vi "PC Controller.vi"() -> ()   [LabVIEW 2017]
panel:
  out "Previous System Status":string
  out "TCP Error Code":i8
  out "Recieved from MyRIO":dbl
  out "TCP Stop Latch":bool
  in  "Send to MyRIO":dbl
  out "System Status":string
  in  "System switch":bool
  in  "MyRIO IP Address":string="localhost"
  out "Current Time":timestamp format="%<%H:%M:%S\n%x>T"
  in  "Logout":bool
  out "Close Event 4 LED":bool
  out "Open Event 4 LED":bool
  out "Close Event 3 LED":bool
  out "Open Event 3 LED":bool
  in  "Close Event Time 4 Edit":timestamp format="%<%H:%M:%S\n%x>T"
  in  "Open Event Time 4 Edit":timestamp format="%<%H:%M:%S\n%x>T"
  in  "Close Event Time 3 Edit":timestamp format="%<%H:%M:%S\n%x>T"
  in  "Open Event Time 3 Edit":timestamp format="%<%H:%M:%S\n%x>T"
  out "Close Event Time 4":timestamp format="%<%H:%M:%S\n%x>T"
  out "Open Event Time 4":timestamp format="%<%H:%M:%S\n%x>T"
  out "Close Event Time 3":timestamp format="%<%H:%M:%S\n%x>T"
  out "Open Event Time 3":timestamp format="%<%H:%M:%S\n%x>T"
  out "Close Event 2 LED":bool
  out "Open Event 2 LED":bool
  out "Close Event 1 LED":bool
  out "Open Event 1 LED":bool
  in  "Close Event Time 2 Edit":timestamp format="%<%H:%M:%S\n%x>T"
  in  "Open Event Time 2 Edit":timestamp format="%<%H:%M:%S\n%x>T"
  in  "Close Event Time 1 Edit":timestamp format="%<%H:%M:%S\n%x>T"
  in  "Open Event Time 1 Edit":timestamp format="%<%H:%M:%S\n%x>T"
  out "Close Event Time 2":timestamp format="%<%H:%M:%S\n%x>T"
  out "Open Event Time 2":timestamp format="%<%H:%M:%S\n%x>T"
  out "Close Event Time 1":timestamp format="%<%H:%M:%S\n%x>T"
  out "Open Event Time 1":timestamp format="%<%H:%M:%S\n%x>T"
  out "Login Attempts":i8
  out "Login Status":string
  in  "Login Button":bool
  in  "Password":string
  in  "Username":string
  out "MyRIO Movement":T1(graph)
  out "Core Temp":dbl format="%#_4g"
  # "Event Time"
  # "Status"
  # "Change Event Time"
  # "On"
  # "Off"
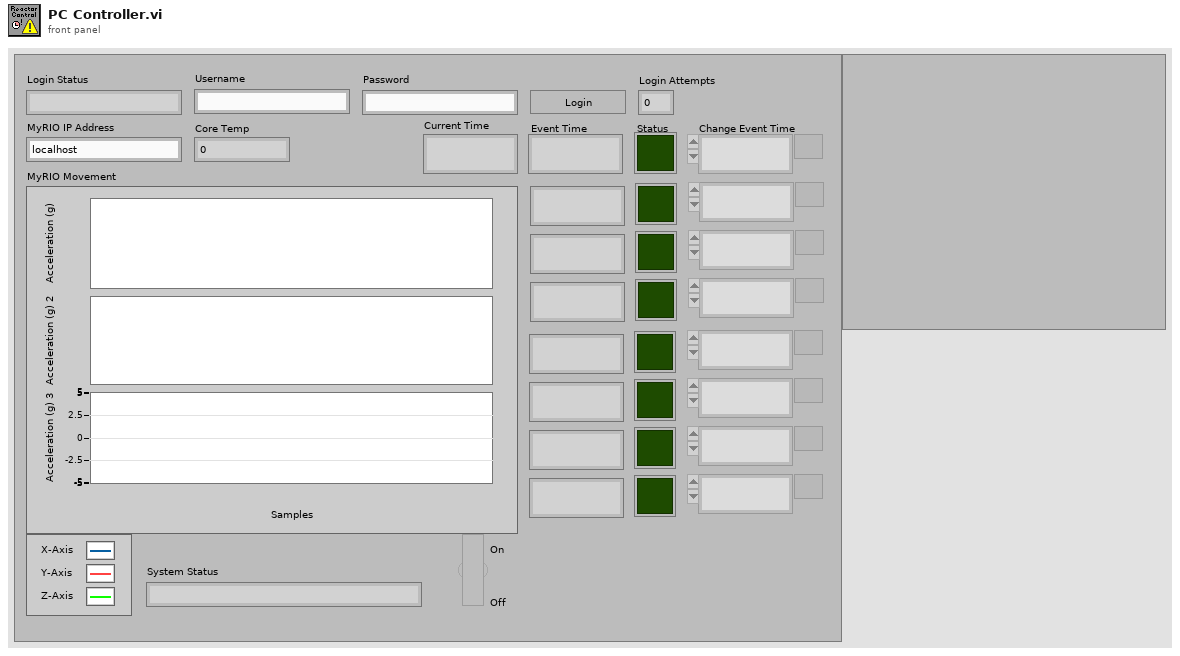
[diagram p1: front panel]
types:
  T1 = cluster{"X-Axis":dbl, "Y-Axis":dbl, "Z-Axis":dbl}
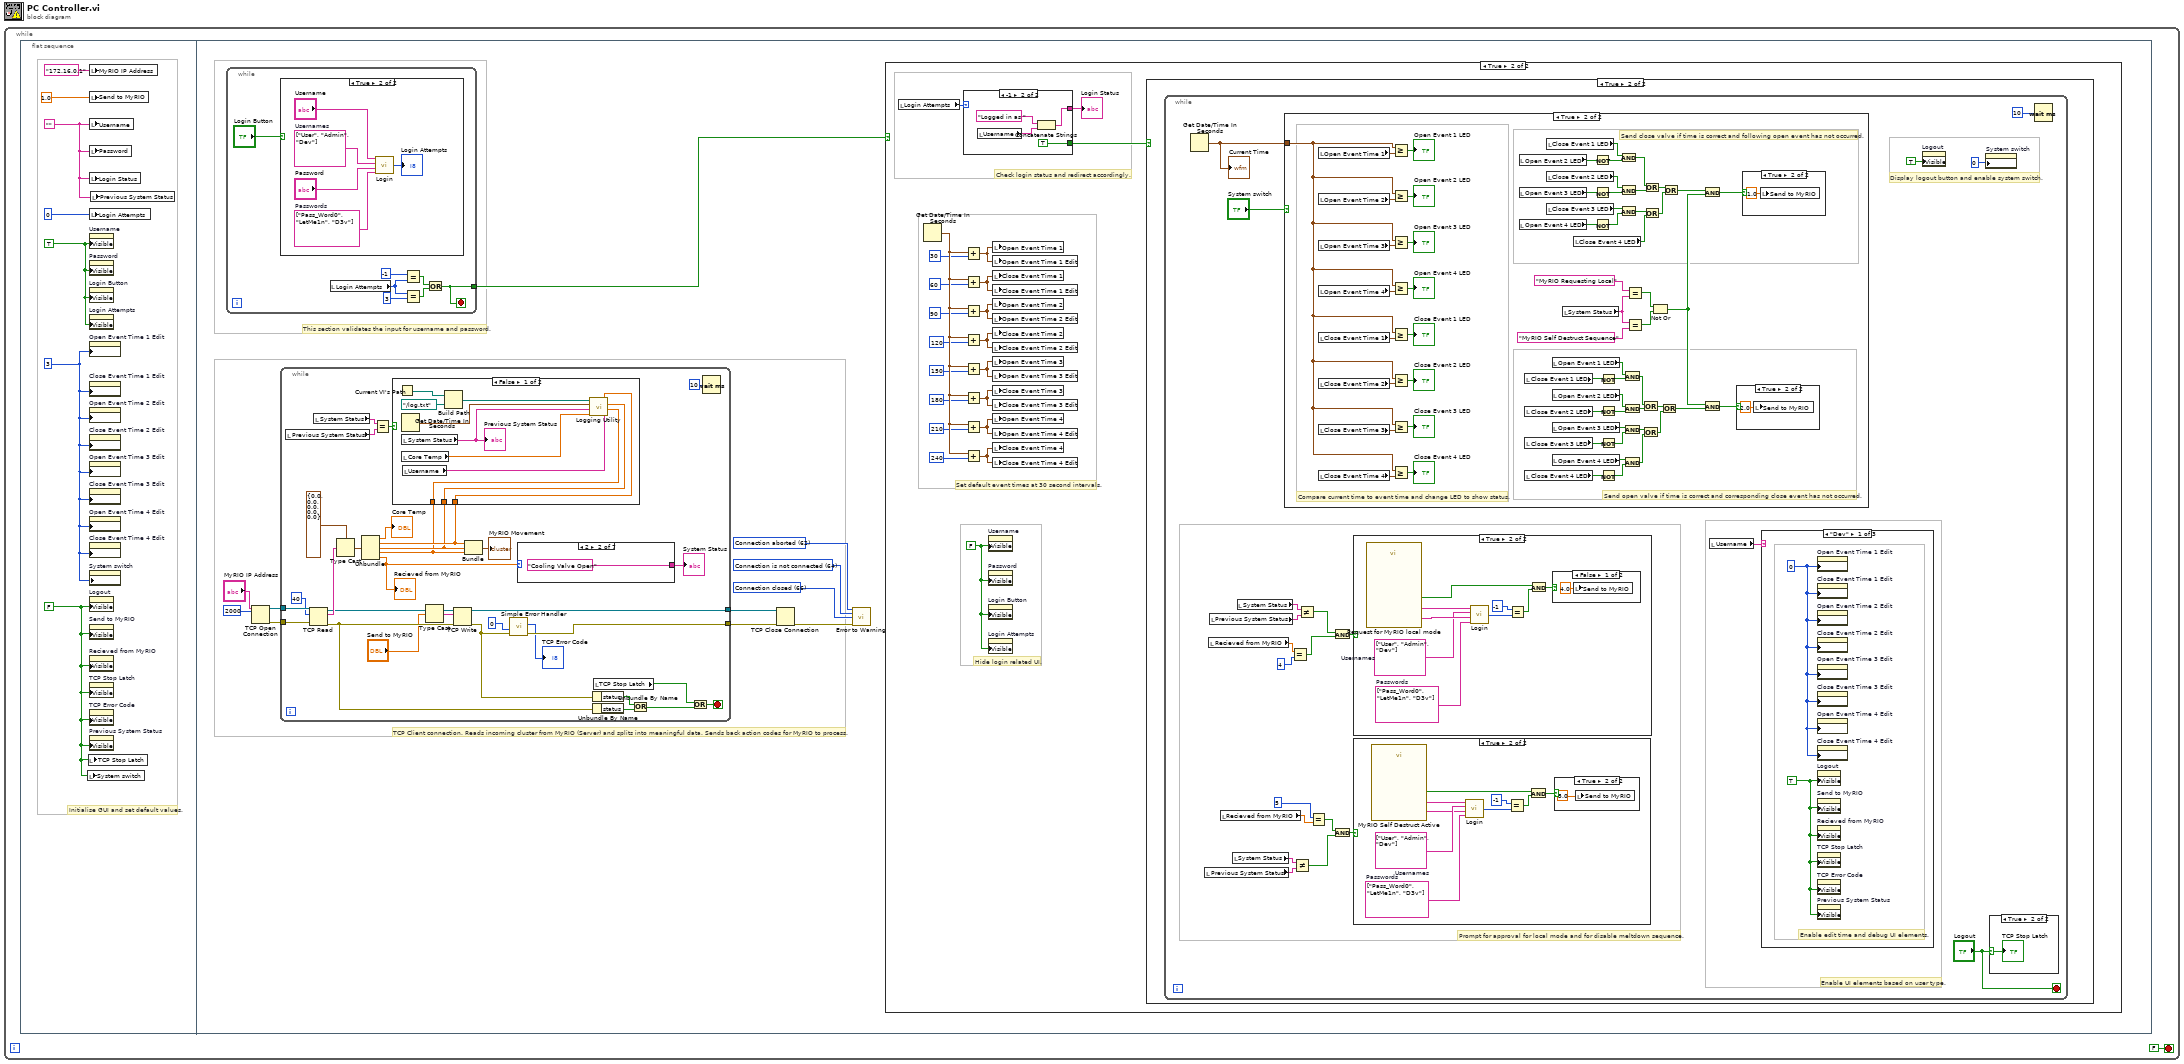
[diagram p0: block diagram]
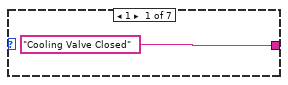
[diagram p3: hidden frame]
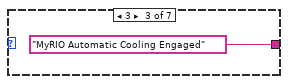
[diagram p4: hidden frame]
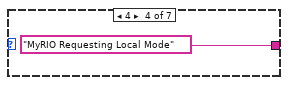
[diagram p5: hidden frame]
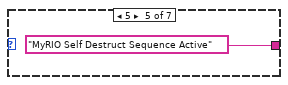
[diagram p6: hidden frame]
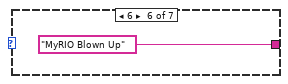
[diagram p7: hidden frame]
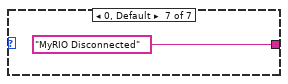
[diagram p8: hidden frame]
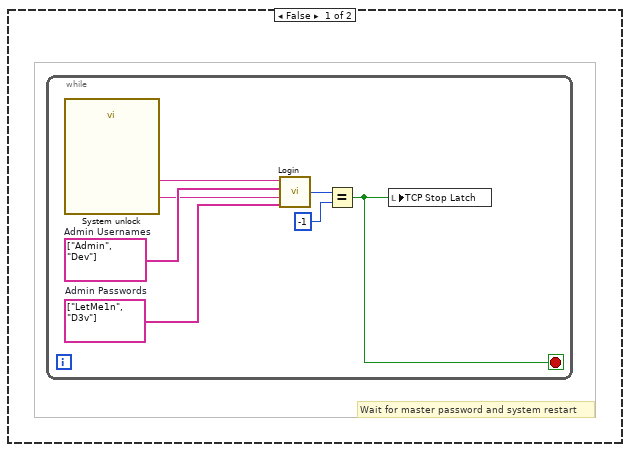
[diagram p10: hidden frame]
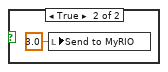
[diagram p14: hidden frame]
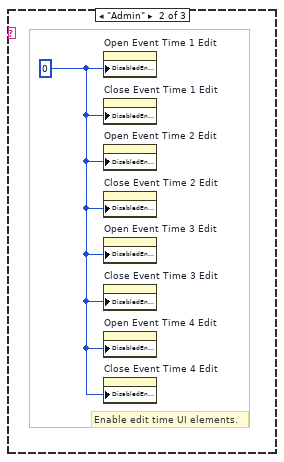
[diagram p15: hidden frame]
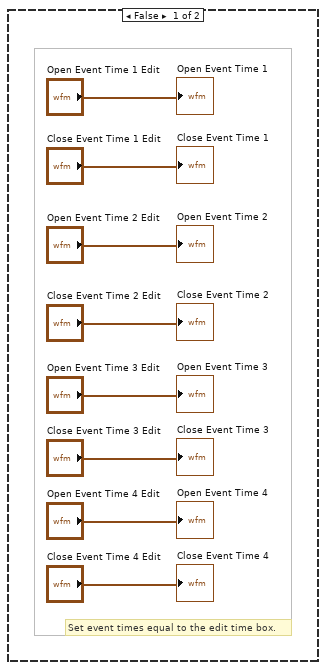
[diagram p17: hidden frame]
diagram:
  n1 = while {
    stop <- FALSE stop-if-true
    n2 = flat-sequence {
      frame #0 {
        w3 = FALSE
        w8 = TRUE
        w7 = 3
        w2 = ""
        # "Initialise GUI and set default values."
        n3 = local write "System switch"(w3) -> ()
        n4 = local write "TCP Stop Latch"(w3) -> ()
        n5 = local write "MyRIO IP Address"("172.16.0.1") -> ()
        n6 = local write "Send to MyRIO"(1.0) -> ()
        n7 = local write "Username"(w2) -> ()
        n8 = local write "Password"(w2) -> ()
        n9 = local write "Login Status"(w2) -> ()
        n10 = local write "Login Attempts"(u32 0 ("milliseconds to wait")) -> ()
        n11 = property on="Username" class="Str"("Visible"=w8) -> ()  [unwired: 2 in, 2 out]
        n12 = property on="Password" class="Str"("Visible"=w8) -> ()  [unwired: 2 in, 2 out]
        n13 = property on="Login Button" class="Bool"("Visible"=w8) -> ()  [unwired: 2 in, 2 out]
        n14 = property on="Login Attempts" class="DigNum (strict)"("Visible"=w8) -> ()  [unwired: 2 in, 2 out]
        n15 = property on="Open Event Time 1 Edit" class="AbsTime (strict)"("DisabledEnum"=w7) -> ()  [unwired: 2 in, 2 out]
        n16 = property on="Close Event Time 1 Edit" class="AbsTime (strict)"("DisabledEnum"=w7) -> ()  [unwired: 2 in, 2 out]
        n17 = property on="Open Event Time 2 Edit" class="AbsTime (strict)"("DisabledEnum"=w7) -> ()  [unwired: 2 in, 2 out]
        n18 = property on="Close Event Time 2 Edit" class="AbsTime (strict)"("DisabledEnum"=w7) -> ()  [unwired: 2 in, 2 out]
        n19 = property on="Open Event Time 3 Edit" class="AbsTime (strict)"("DisabledEnum"=w7) -> ()  [unwired: 2 in, 2 out]
        n20 = property on="Close Event Time 3 Edit" class="AbsTime (strict)"("DisabledEnum"=w7) -> ()  [unwired: 2 in, 2 out]
        n21 = property on="Open Event Time 4 Edit" class="AbsTime (strict)"("DisabledEnum"=w7) -> ()  [unwired: 2 in, 2 out]
        n22 = property on="Close Event Time 4 Edit" class="AbsTime (strict)"("DisabledEnum"=w7) -> ()  [unwired: 2 in, 2 out]
        n23 = property on="Logout" class="Bool"("Visible"=w3) -> ()  [unwired: 2 in, 2 out]
        n24 = property on="Send to MyRIO" class="DigNum (strict)"("Visible"=w3) -> ()  [unwired: 2 in, 2 out]
        n25 = property on="Recieved from MyRIO" class="DigNum (strict)"("Visible"=w3) -> ()  [unwired: 2 in, 2 out]
        n26 = property on="TCP Stop Latch" class="Bool (strict)"("Visible"=w3) -> ()  [unwired: 2 in, 2 out]
        n27 = property on="TCP Error Code" class="DigNum (strict)"("Visible"=w3) -> ()  [unwired: 2 in, 2 out]
        n28 = property on="Previous System Status" class="Str"("Visible"=w3) -> ()  [unwired: 2 in, 2 out]
        n29 = property on="System switch" class="Bool (strict)"("DisabledEnum"=w7) -> ()  [unwired: 2 in, 2 out]
        n30 = local write "Previous System Status"(w2) -> ()
      }
      frame #1 {
        w9 = 66 items=["No Error", "Argument Error", "Memory Full", "Out of Zone", "End of File", "File Already Open", "Generic File IO Error", "File Not Found", "File Permission Error", "Disk Full", "Duplicate Path", "Too Many Files Open", "Not Enabled", "Resource File Not Found", "Cannot Add Resource", "Resource Not Found", "Image Not Found", "Image Memory Error", "Pen Does Not Exist", "Config Bad Type", "Config Token Not Found", "Config Parse Error", "Config Memory Error", "Bad External Code Format", "Bad External Code Offset", "External Code Not Present", "Null Window", "Destroy Window Mixup", "Null Menu", "Print Aborted", "Bad Print Record", "Print Driver Error", "Windows Error During Print", "Memory Error During Print", "Print Dialog Error", "Generic Print Error", "Invalid Device Refnum", "Device Not Found", "Device Parameter Error", "Device Unit Error", "Can't Open Device", "Device Call Aborted", "Generic Error", "Cancelled By User", "Object ID Too Low", "Object ID Too High", "Object Not In Heap", "Unknown Heap", "Bad DefProc ID", "DefProc Not In Table", "Message Out Of Range", "Null Method", "Unknown Message", "Manager Call Not Supported", "Bad address", "Connection In progress", "Connection timed out", "Connection is already in progress", "Network attribute not supported", "Network error", "Address in use", "System out of memory", "Connection aborted", "Connection refused", "Connection is not connected", "Connection is already connected", "Connection closed", "Initialize error (interapplication manager)", "Bad occurrence", "Wait on unbound occurrence handler", "Occurrence queue overflow", "Bad path", "Semaphore not signaled", "Unrecognized type (interapplication manager)"] ("1st Error to Convert")
        w10 = 64 items=["No Error", "Argument Error", "Memory Full", "Out of Zone", "End of File", "File Already Open", "Generic File IO Error", "File Not Found", "File Permission Error", "Disk Full", "Duplicate Path", "Too Many Files Open", "Not Enabled", "Resource File Not Found", "Cannot Add Resource", "Resource Not Found", "Image Not Found", "Image Memory Error", "Pen Does Not Exist", "Config Bad Type", "Config Token Not Found", "Config Parse Error", "Config Memory Error", "Bad External Code Format", "Bad External Code Offset", "External Code Not Present", "Null Window", "Destroy Window Mixup", "Null Menu", "Print Aborted", "Bad Print Record", "Print Driver Error", "Windows Error During Print", "Memory Error During Print", "Print Dialog Error", "Generic Print Error", "Invalid Device Refnum", "Device Not Found", "Device Parameter Error", "Device Unit Error", "Can't Open Device", "Device Call Aborted", "Generic Error", "Cancelled By User", "Object ID Too Low", "Object ID Too High", "Object Not In Heap", "Unknown Heap", "Bad DefProc ID", "DefProc Not In Table", "Message Out Of Range", "Null Method", "Unknown Message", "Manager Call Not Supported", "Bad address", "Connection In progress", "Connection timed out", "Connection is already in progress", "Network attribute not supported", "Network error", "Address in use", "System out of memory", "Connection aborted", "Connection refused", "Connection is not connected", "Connection is already connected", "Connection closed", "Initialize error (interapplication manager)", "Bad occurrence", "Wait on unbound occurrence handler", "Occurrence queue overflow", "Bad path", "Semaphore not signaled", "Unrecognized type (interapplication manager)"] ("1st Error to Convert")
        w11 = 62 items=["No Error", "Argument Error", "Memory Full", "Out of Zone", "End of File", "File Already Open", "Generic File IO Error", "File Not Found", "File Permission Error", "Disk Full", "Duplicate Path", "Too Many Files Open", "Not Enabled", "Resource File Not Found", "Cannot Add Resource", "Resource Not Found", "Image Not Found", "Image Memory Error", "Pen Does Not Exist", "Config Bad Type", "Config Token Not Found", "Config Parse Error", "Config Memory Error", "Bad External Code Format", "Bad External Code Offset", "External Code Not Present", "Null Window", "Destroy Window Mixup", "Null Menu", "Print Aborted", "Bad Print Record", "Print Driver Error", "Windows Error During Print", "Memory Error During Print", "Print Dialog Error", "Generic Print Error", "Invalid Device Refnum", "Device Not Found", "Device Parameter Error", "Device Unit Error", "Can't Open Device", "Device Call Aborted", "Generic Error", "Cancelled By User", "Object ID Too Low", "Object ID Too High", "Object Not In Heap", "Unknown Heap", "Bad DefProc ID", "DefProc Not In Table", "Message Out Of Range", "Null Method", "Unknown Message", "Manager Call Not Supported", "Bad address", "Connection In progress", "Connection timed out", "Connection is already in progress", "Network attribute not supported", "Network error", "Address in use", "System out of memory", "Connection aborted", "Connection refused", "Connection is not connected", "Connection is already connected", "Connection closed", "Initialize error (interapplication manager)", "Bad occurrence", "Wait on unbound occurrence handler", "Occurrence queue overflow", "Bad path", "Semaphore not signaled", "Unrecognized type (interapplication manager)"] ("1st Error to Convert")
        # "TCP Client connection. Reads incoming cluster from MyRIO (Server) and splits into meaningful data. Sends back action codes for MyRIO to process."
        # "This section validates the input for username and password."
        n31 = while {
          tunnel: [w218] -> w19
          stop <- w218 stop-if-true
          n32 = case shown="True" "Login Button" {
            frame False {
            }
            frame True {
              w226 = string[] ["Pass_Word0", "LetMe1n", "D3v"]  # Passwords
              w228 = string[] ["User", "Admin", "Dev"]  # Usernames
              n33 = call "Login.vi"("Passwords"=w226, "Password"="Password", "Usernames"=w228, "Username"="Username") -> ("Login Attempts"=→"Login Attempts":i8)
            }
          }
          n34 = local read "Login Attempts"() -> (w221:i8)
          n35 = Equal?(x=-1, y=w221) -> (x = y?=w220:bool)
          n36 = Equal?(x=w221, y=3) -> (x = y?=w219:bool)
          n37 = Or(x=w220, y=w219) -> (x .or. y?=w218:bool)
        }
        n38 = TCP Open Connection(address="MyRIO IP Address", remote port or service name=u16 2000) -> (connection ID=w14:refnum<k5>, error out=w15:errorcluster)  [unwired: 1 in, 2 out]
        n39 = while {
          tunnel: w15 -> [w50]
          tunnel: w14 -> [w49]
          tunnel: [w32] -> w17
          tunnel: [w33] -> w18
          stop <- w37 stop-if-true
          n40 = local read "Previous System Status"() -> (w25:string)
          n41 = TCP Read(connection ID=w49, bytes to read=40, error in (no error)=w50) -> (connection ID out=w42:refnum<k5>, data out=w47:string, error out=w41:errorcluster)  [unwired: 2 in]
          n42 = local read "System Status"() -> (w26:string)
          n43 = Type Cast(type=cluster{dbl, dbl, dbl, dbl, dbl} {0.0, 0.0, 0.0, 0.0, 0.0}, x=w47) -> (*(type *) &x=w45:cluster{dbl, dbl, dbl, dbl, dbl})
          n44 = Unbundle(w45) -> (→"Core Temp":dbl, w22:dbl, w21:dbl, w20:dbl, w27:dbl)
          "Recieved from MyRIO" <- w27
          n45 = Equal?(x=w26, y=w25) -> (x = y?=w24:bool)
          n46 = case shown="False" w24 {
            tunnel: w22 -> [w53 _]
            tunnel: w21 -> [w52 _]
            tunnel: w20 -> [w51 _]
            frame False {
              n47 = Current VI's Path() -> (path=w60:path)
              n48 = Get Date/Time In Seconds() -> (seconds since 1Jan1904=w55:timestamp)
              n49 = local read "System Status"() -> (w57:string)
              "Previous System Status" <- w57
              n50 = local read "Core Temp"() -> (w54:dbl)
              n51 = local read "Username"() -> (w56:string)
              n52 = Build Path(base path=w60, name or relative path=path "../log.txt") -> (appended path=w58:path)
              n53 = call "Logging Utility.vi"("Username"=w56, "Z Coord"=w51, "Y Coord"=w52, "X Coord"=w53, "Temperature"=w54, "Event"=w57, "Timestamp"=w55, "Path"=w58) -> ()
            }
            frame True {
            }
          }
          n54 = Type Cast(x="Send to MyRIO") -> (*(type *) &x=w40:string)  [unwired: 1 in]
          n55 = TCP Write(connection ID=w42, data in=w40, error in (no error)=w41) -> (connection ID out=w33:refnum<k5>, error out=w31:errorcluster)  [unwired: 1 in, 1 out]
          n56 = Bundle(w22, w21, w20) -> (→"MyRIO Movement":cluster{dbl, dbl, dbl})  [unwired: 1 in]
          n57 = call <vilib>:"Simple Error Handler.vi"("type of dialog (OK msg:1)"=u32 0 ("milliseconds to wait"), "error in (no error)"=w31) -> ("code out"=→"TCP Error Code":i32, "error out"=w32:errorcluster)  [unwired: 3 in, 3 out]
          n58 = case shown="2" w27 {
            tunnel: ["Cooling Valve Closed" "Cooling Valve Open" "MyRIO Automatic Cooling Engaged" "MyRIO Requesting Local Mode" "MyRIO Self Destruct Sequence Active" "MyRIO Blown Up" "MyRIO Disconnected"] -> w28
            frame 1 {
            }
            frame 2 {
            }
            frame 3 {
            }
            frame 4 {
            }
            frame 5 {
            }
            frame 6 {
            }
            frame 0, Default {
            }
          }
          "System Status" <- w28
          n59 = Unbundle By Name(w31) -> ("status"=w38:bool)
          n60 = Unbundle By Name(w41) -> ("status"=w39:bool)
          n61 = local read "TCP Stop Latch"() -> (w35:bool)
          n62 = Or(x=w38, y=w39) -> (x .or. y?=w36:bool)
          n63 = Or(x=w35, y=w36) -> (x .or. y?=w37:bool)
          n64 = Wait (ms)(milliseconds to wait=u32 10) -> ()  [unwired: 1 out]
        }
        n65 = TCP Close Connection(connection ID=w18, error in (no error)=w17) -> (error out=w12:errorcluster)  [unwired: 1 in, 1 out]
        n66 = call <vilib>:"Error to Warning.vi"("1st Error to Convert"=w11, "2nd Error to Convert"=w10, "3rd Error to Convert"=w9, "error in"=w12) -> ()  [unwired: 2 in, 10 out]
        n67 = case shown="True" w19 {
          frame False {
          }
          frame True {
            w86 = FALSE
            # "Set default event times at 30 second intervals."
            # "Hide login related UI."
            # "Check login status and redirect accordingly."
            n68 = local read "Login Attempts"() -> (w88:i8)
            n69 = Get Date/Time In Seconds() -> (seconds since 1Jan1904=w76:timestamp)
            n70 = case shown="-1" w88 {
              tunnel: ["Bad login, system locked  " w216] -> w87
              tunnel: [FALSE TRUE] -> w85
              frame 3, Default {
              }
              frame -1 {
                n71 = local read "Username"() -> (w215:string)
                n72 = Concatenate Strings("Logged in as ", w215) -> (w216:string)
              }
            }
            "Login Status" <- w87
            n73 = Add(x=w76, y=30) -> (x+y=w77:timestamp)
            n74 = Add(x=w76, y=60) -> (x+y=w78:timestamp)
            n75 = Add(x=w76, y=90) -> (x+y=w79:timestamp)
            n76 = Add(x=w76, y=120) -> (x+y=w80:timestamp)
            n77 = Add(x=w76, y=150) -> (x+y=w81:timestamp)
            n78 = Add(x=w76, y=180) -> (x+y=w82:timestamp)
            n79 = Add(x=w76, y=210) -> (x+y=w83:timestamp)
            n80 = Add(x=w76, y=240) -> (x+y=w84:timestamp)
            n81 = property on="Username" class="Str"("Visible"=w86) -> ()  [unwired: 2 in, 2 out]
            n82 = property on="Password" class="Str"("Visible"=w86) -> ()  [unwired: 2 in, 2 out]
            n83 = property on="Login Button" class="Bool"("Visible"=w86) -> ()  [unwired: 2 in, 2 out]
            n84 = property on="Login Attempts" class="DigNum (strict)"("Visible"=w86) -> ()  [unwired: 2 in, 2 out]
            n85 = local write "Open Event Time 1"(w77) -> ()
            n86 = local write "Open Event Time 1 Edit"(w77) -> ()
            n87 = local write "Close Event Time 1"(w78) -> ()
            n88 = local write "Close Event Time 1 Edit"(w78) -> ()
            n89 = local write "Open Event Time 2"(w79) -> ()
            n90 = local write "Open Event Time 2 Edit"(w79) -> ()
            n91 = local write "Close Event Time 2"(w80) -> ()
            n92 = local write "Close Event Time 2 Edit"(w80) -> ()
            n93 = local write "Open Event Time 3"(w81) -> ()
            n94 = local write "Open Event Time 3 Edit"(w81) -> ()
            n95 = local write "Close Event Time 3"(w82) -> ()
            n96 = local write "Close Event Time 3 Edit"(w82) -> ()
            n97 = local write "Open Event Time 4"(w83) -> ()
            n98 = local write "Open Event Time 4 Edit"(w83) -> ()
            n99 = local write "Close Event Time 4"(w84) -> ()
            n100 = local write "Close Event Time 4 Edit"(w84) -> ()
            n101 = case shown="True" w85 {
              frame False {
                # "Wait for master password and system restart"
                n102 = while {
                  stop <- w89 stop-if-true
                  w92 = string[] ["LetMe1n", "D3v"]  # Admin Passwords
                  w94 = string[] ["Admin", "Dev"]  # Admin Usernames
                  n103 = call "System unlock"() -> ("Password"=w93:string, "Username"=w95:string)  [unwired: 16 in, 2 out]
                  n104 = call "Login.vi"("Passwords"=w92, "Password"=w93, "Usernames"=w94, "Username"=w95) -> ("Login Attempts"=w91:i8)
                  n105 = Equal?(x=w91, y=-1) -> (x = y?=w89:bool)
                  n106 = local write "TCP Stop Latch"(w89) -> ()
                }
              }
              frame True {
                n107 = while {
                  stop <- "Logout" stop-if-true
                  # "Prompt for approval for local mode and for disable meltdown sequence."
                  # "Enable UI elements based on user type."
                  # "Display logout button and enable system switch."
                  n108 = Get Date/Time In Seconds() -> (seconds since 1Jan1904=w113:timestamp)
                  "Current Time" <- w113
                  n109 = local read "Previous System Status"() -> (w105:string)
                  n110 = local read "Recieved from MyRIO"() -> (w101:dbl)
                  n111 = local read "Previous System Status"() -> (w108:string)
                  n112 = local read "Recieved from MyRIO"() -> (w97:dbl)
                  n113 = local read "System Status"() -> (w104:string)
                  n114 = local read "System Status"() -> (w109:string)
                  n115 = case shown="True" "System switch" {
                    tunnel: w113 -> [_ w159]
                    frame False {
                      # "Set event times equal to the edit time box."
                      "Close Event Time 1" <- "Close Event Time 1 Edit"
                      "Open Event Time 2" <- "Open Event Time 2 Edit"
                      "Close Event Time 2" <- "Close Event Time 2 Edit"
                      "Open Event Time 1" <- "Open Event Time 1 Edit"
                      "Open Event Time 3" <- "Open Event Time 3 Edit"
                      "Close Event Time 3" <- "Close Event Time 3 Edit"
                      "Open Event Time 4" <- "Open Event Time 4 Edit"
                      "Close Event Time 4" <- "Close Event Time 4 Edit"
                    }
                    frame True {
                      # "Compare current time to event time and change LED to show status."
                      # "Send close valve if time is correct and following open event has not occurred."
                      # "Send open valve if time is correct and corresponding close event has not occurred."
                      n116 = local read "Open Event Time 1"() -> (w202:timestamp)
                      n117 = local read "Open Event Time 2"() -> (w208:timestamp)
                      n118 = local read "Open Event Time 3"() -> (w206:timestamp)
                      n119 = local read "Open Event Time 4"() -> (w204:timestamp)
                      n120 = local read "Close Event Time 1"() -> (w201:timestamp)
                      n121 = local read "Close Event Time 2"() -> (w207:timestamp)
                      n122 = local read "Close Event Time 3"() -> (w205:timestamp)
                      n123 = local read "Close Event Time 4"() -> (w203:timestamp)
                      n124 = Greater Or Equal?(x=w159, y=w202) -> (x >= y?=→"Open Event 1 LED":bool)
                      n125 = Greater Or Equal?(x=w159, y=w208) -> (x >= y?=→"Open Event 2 LED":bool)
                      n126 = Greater Or Equal?(x=w159, y=w206) -> (x >= y?=→"Open Event 3 LED":bool)
                      n127 = Greater Or Equal?(x=w159, y=w204) -> (x >= y?=→"Open Event 4 LED":bool)
                      n128 = Greater Or Equal?(x=w159, y=w201) -> (x >= y?=→"Close Event 1 LED":bool)
                      n129 = Greater Or Equal?(x=w159, y=w207) -> (x >= y?=→"Close Event 2 LED":bool)
                      n130 = Greater Or Equal?(x=w159, y=w205) -> (x >= y?=→"Close Event 3 LED":bool)
                      n131 = Greater Or Equal?(x=w159, y=w203) -> (x >= y?=→"Close Event 4 LED":bool)
                      n132 = local read "Open Event 2 LED"() -> (w178:bool)
                      n133 = local read "Open Event 3 LED"() -> (w179:bool)
                      n134 = local read "Open Event 4 LED"() -> (w180:bool)
                      n135 = local read "Close Event 1 LED"() -> (w162:bool)
                      n136 = local read "Close Event 2 LED"() -> (w163:bool)
                      n137 = local read "Close Event 3 LED"() -> (w164:bool)
                      n138 = local read "Close Event 4 LED"() -> (w165:bool)
                      n139 = local read "Close Event 1 LED"() -> (w186:bool)
                      n140 = local read "Close Event 2 LED"() -> (w184:bool)
                      n141 = local read "Close Event 3 LED"() -> (w182:bool)
                      n142 = local read "Open Event 1 LED"() -> (w168:bool)
                      n143 = local read "Open Event 2 LED"() -> (w169:bool)
                      n144 = local read "Open Event 3 LED"() -> (w170:bool)
                      n145 = local read "Open Event 4 LED"() -> (w171:bool)
                      n146 = local read "System Status"() -> (w158:string)
                      n147 = local read "Close Event 4 LED"() -> (w191:bool)
                      n148 = Not(x=w178) -> (.not. x?=w185:bool)
                      n149 = Not(x=w179) -> (.not. x?=w183:bool)
                      n150 = Not(x=w180) -> (.not. x?=w181:bool)
                      n151 = Not(x=w162) -> (.not. x?=w160:bool)
                      n152 = Not(x=w163) -> (.not. x?=w161:bool)
                      n153 = Not(x=w164) -> (.not. x?=w166:bool)
                      n154 = Not(x=w165) -> (.not. x?=w167:bool)
                      n155 = And(x=w186, y=w185) -> (x .and. y?=w187:bool)
                      n156 = And(x=w184, y=w183) -> (x .and. y?=w188:bool)
                      n157 = And(x=w182, y=w181) -> (x .and. y?=w190:bool)
                      n158 = And(x=w168, y=w160) -> (x .and. y?=w172:bool)
                      n159 = And(x=w169, y=w161) -> (x .and. y?=w173:bool)
                      n160 = And(x=w170, y=w166) -> (x .and. y?=w174:bool)
                      n161 = And(x=w171, y=w167) -> (x .and. y?=w175:bool)
                      n162 = Equal?(x="MyRIO Requesting Local", y=w158) -> (x = y?=w155:bool)
                      n163 = Equal?(x=w158, y="MyRIO Self Destruct Sequence") -> (x = y?=w154:bool)
                      n164 = Or(x=w172, y=w173) -> (x .or. y?=w177:bool)
                      n165 = Or(x=w174, y=w175) -> (x .or. y?=w176:bool)
                      n166 = Or(x=w187, y=w188) -> (x .or. y?=w189:bool)
                      n167 = Or(x=w190, y=w191) -> (x .or. y?=w192:bool)
                      n168 = Not Or(1:w154, 2:w155) -> (0:w151:bool)
                      n169 = Or(x=w177, y=w176) -> (x .or. y?=w150:bool)
                      n170 = Or(x=w189, y=w192) -> (x .or. y?=w153:bool)
                      n171 = And(x=w153, y=w151) -> (x .and. y?=w152:bool)
                      n172 = And(x=w151, y=w150) -> (x .and. y?=w149:bool)
                      n173 = case shown="True" w149 {
                        frame False {
                        }
                        frame True {
                          n174 = local write "Send to MyRIO"(2.0) -> ()
                        }
                      }
                      n175 = case shown="True" w152 {
                        frame False {
                        }
                        frame True {
                          n176 = local write "Send to MyRIO"(1.0) -> ()
                        }
                      }
                    }
                  }
                  n177 = Equal?(x=w101, y=4) -> (x = y?=w99:bool)
                  n178 = Not Equal?(x=w104, y=w105) -> (x != y?=w103:bool)
                  n179 = Not Equal?(x=w109, y=w108) -> (x != y?=w102:bool)
                  n180 = Equal?(x=5, y=w97) -> (x = y?=w98:bool)
                  n181 = And(x=w102, y=w99) -> (x .and. y?=w107:bool)
                  n182 = And(x=w98, y=w103) -> (x .and. y?=w106:bool)
                  n183 = case shown="True" w106 {
                    frame False {
                    }
                    frame True {
                      w122 = string[] ["Pass_Word0", "LetMe1n", "D3v"]  # Passwords
                      w123 = string[] ["User", "Admin", "Dev"]  # Usernames
                      n184 = call "MyRIO Self Destruct Active"() -> ("Password"=w118:string, "Username"=w119:string, "Submit"=w117:bool)  [unwired: 16 in, 1 out]
                      n185 = call "Login.vi"("Passwords"=w122, "Password"=w118, "Usernames"=w123, "Username"=w119) -> ("Login Attempts"=w121:i8)
                      n186 = Equal?(x=-1, y=w121) -> (x = y?=w124:bool)
                      n187 = And(x=w117, y=w124) -> (x .and. y?=w120:bool)
                      n188 = case shown="True" w120 {
                        frame False {
                        }
                        frame True {
                          n189 = local write "Send to MyRIO"(5.0) -> ()
                        }
                      }
                    }
                  }
                  n190 = case shown="True" w107 {
                    frame False {
                    }
                    frame True {
                      w130 = string[] ["Pass_Word0", "LetMe1n", "D3v"]  # Passwords
                      w131 = string[] ["User", "Admin", "Dev"]  # Usernames
                      n191 = call "Request for MyRIO local mode"() -> ("Password"=w134:string, "Username"=w135:string, "Approve"=w127:bool)  [unwired: 16 in, 1 out]
                      n192 = call "Login.vi"("Passwords"=w130, "Password"=w134, "Usernames"=w131, "Username"=w135) -> ("Login Attempts"=w129:i8)
                      n193 = Equal?(x=-1, y=w129) -> (x = y?=w132:bool)
                      n194 = And(x=w127, y=w132) -> (x .and. y?=w128:bool)
                      n195 = case shown="False" w128 {
                        frame False {
                          n196 = local write "Send to MyRIO"(4.0) -> ()
                        }
                        frame True {
                          n197 = local write "Send to MyRIO"(3.0) -> ()
                        }
                      }
                    }
                  }
                  n198 = local read "Username"() -> (w110:string)
                  n199 = case shown="\"Dev\"" w110 {
                    frame "Dev" {
                      w138 = TRUE
                      w139 = 0
                      # "Enable edit time and debug UI elements."
                      n200 = property on="Open Event Time 1 Edit" class="AbsTime (strict)"("DisabledEnum"=w139) -> ()  [unwired: 2 in, 2 out]
                      n201 = property on="Close Event Time 1 Edit" class="AbsTime (strict)"("DisabledEnum"=w139) -> ()  [unwired: 2 in, 2 out]
                      n202 = property on="Open Event Time 2 Edit" class="AbsTime (strict)"("DisabledEnum"=w139) -> ()  [unwired: 2 in, 2 out]
                      n203 = property on="Close Event Time 2 Edit" class="AbsTime (strict)"("DisabledEnum"=w139) -> ()  [unwired: 2 in, 2 out]
                      n204 = property on="Open Event Time 3 Edit" class="AbsTime (strict)"("DisabledEnum"=w139) -> ()  [unwired: 2 in, 2 out]
                      n205 = property on="Close Event Time 3 Edit" class="AbsTime (strict)"("DisabledEnum"=w139) -> ()  [unwired: 2 in, 2 out]
                      n206 = property on="Open Event Time 4 Edit" class="AbsTime (strict)"("DisabledEnum"=w139) -> ()  [unwired: 2 in, 2 out]
                      n207 = property on="Close Event Time 4 Edit" class="AbsTime (strict)"("DisabledEnum"=w139) -> ()  [unwired: 2 in, 2 out]
                      n208 = property on="Logout" class="Bool"("Visible"=w138) -> ()  [unwired: 2 in, 2 out]
                      n209 = property on="Send to MyRIO" class="DigNum (strict)"("Visible"=w138) -> ()  [unwired: 2 in, 2 out]
                      n210 = property on="Recieved from MyRIO" class="DigNum (strict)"("Visible"=w138) -> ()  [unwired: 2 in, 2 out]
                      n211 = property on="TCP Stop Latch" class="Bool (strict)"("Visible"=w138) -> ()  [unwired: 2 in, 2 out]
                      n212 = property on="TCP Error Code" class="DigNum (strict)"("Visible"=w138) -> ()  [unwired: 2 in, 2 out]
                      n213 = property on="Previous System Status" class="Str"("Visible"=w138) -> ()  [unwired: 2 in, 2 out]
                    }
                    frame "Admin" {
                      w140 = 0
                      # "Enable edit time UI elements."
                      n214 = property on="Open Event Time 1 Edit" class="AbsTime (strict)"("DisabledEnum"=w140) -> ()  [unwired: 2 in, 2 out]
                      n215 = property on="Close Event Time 1 Edit" class="AbsTime (strict)"("DisabledEnum"=w140) -> ()  [unwired: 2 in, 2 out]
                      n216 = property on="Open Event Time 2 Edit" class="AbsTime (strict)"("DisabledEnum"=w140) -> ()  [unwired: 2 in, 2 out]
                      n217 = property on="Close Event Time 2 Edit" class="AbsTime (strict)"("DisabledEnum"=w140) -> ()  [unwired: 2 in, 2 out]
                      n218 = property on="Open Event Time 3 Edit" class="AbsTime (strict)"("DisabledEnum"=w140) -> ()  [unwired: 2 in, 2 out]
                      n219 = property on="Close Event Time 3 Edit" class="AbsTime (strict)"("DisabledEnum"=w140) -> ()  [unwired: 2 in, 2 out]
                      n220 = property on="Open Event Time 4 Edit" class="AbsTime (strict)"("DisabledEnum"=w140) -> ()  [unwired: 2 in, 2 out]
                      n221 = property on="Close Event Time 4 Edit" class="AbsTime (strict)"("DisabledEnum"=w140) -> ()  [unwired: 2 in, 2 out]
                    }
                    frame Default {
                    }
                  }
                  n222 = property on="Logout" class="Bool"("Visible"=TRUE) -> ()  [unwired: 2 in, 2 out]
                  n223 = property on="System switch" class="Bool (strict)"("DisabledEnum"=0) -> ()  [unwired: 2 in, 2 out]
                  n224 = case shown="True" "Logout" {
                    selector: "Logout" -> [_ w211]
                    frame False {
                    }
                    frame True {
                      "TCP Stop Latch" <- w211
                    }
                  }
                  n225 = Wait (ms)(milliseconds to wait=u32 10) -> ()  [unwired: 1 out]
                }
              }
            }
          }
        }
      }
    }
  }
